vi "DIO_PWM_Encoder_SPI.vi"(0 "DIO.3:0.OUT":fxp<+,4,4> format="%.0b", 1 "DIO.3:0.DIR":fxp<+,4,4> format="%.0b", 2 "PWM.1:0.GROUP IN":T2 {"PWM.1.CNFG" format="%08b"; "PWM.0.CNFG" format="%08b"}, 3 "PWM.3:2.GROUP IN":T2 {"PWM.1.CNFG" format="%08b"; "PWM.0.CNFG" format="%08b"}, 4 "Encoder.0.GROUP IN":T1 {"ENC.STAT" format="%08b"}, 5 "Encoder.1.GROUP IN":T1 {"ENC.STAT" format="%08b"}, 6 "DIO0/PWM0/ENC0.A Refnum":refnum<k21>, 7 "DIO.3:0.Selector":fxp<+,8,8> format="%.0b", 8 "DIO1/PWM1/ENC0.B/SPI.CLK Refnum":refnum<k21>, 9 "SPI.GROUP IN":T3={"SPI.STAT"=0, "SPI.GO"=FALSE, "SPI.CNT"=19, "SPI.CNFG"=112, "SPI.DATI"=0, "SPI.DATO"=0} {"SPI.STAT" format="%08b"}, 10 "DIO2/PWM2/ENC1.A/SPI.MISO Refnum":refnum<k21>, 12 "DIO3/PWM3/ENC1.B/SPI.MOSI Refnum":refnum<k21>) -> (11 "SPI.GROUP OUT":T3={"SPI.STAT"=0, "SPI.GO"=FALSE, "SPI.CNT"=19, "SPI.CNFG"=112, "SPI.DATI"=0, "SPI.DATO"=0} {"SPI.STAT" format="%08b"}, 14 "IN 3:0":fxp<+,4,4> format="%02b", 16 "PWM.1:0.GROUP OUT":T2 {"PWM.1.CNFG" format="%08b"; "PWM.0.CNFG" format="%08b"}, 17 "PWM.3:2.GROUP OUT":T2 {"PWM.1.CNFG" format="%08b"; "PWM.0.CNFG" format="%08b"}, 18 "Encoder.0.GROUP OUT":T1 {"ENC.STAT" format="%08b"}, 19 "Encoder.1.GROUP OUT":T1 {"ENC.STAT" format="%08b"})   [LabVIEW 2021]
uses:
  Utilities/PWM Configuration Group.ctl
  Utilities/Encoder Configuration Group.ctl
  Utilities/Start Boolean.ctl
  Utilities/SPI Configuration Group.ctl
panel:
  # "This VI switches between the DIO functionality and the PWM/Encoder/SPI functionality for the specified FPGA I/O channels. Each bit has a selector which contains two-bits booleans.\n- If SELECT 0 is 00, DIO are enabled.\n- If SELECT 0 is 01, PWM enabled.\n- If SELECT 0 is 10, Encoder enabled.\n- If SELECT 0 is 11, SPI is enabled."
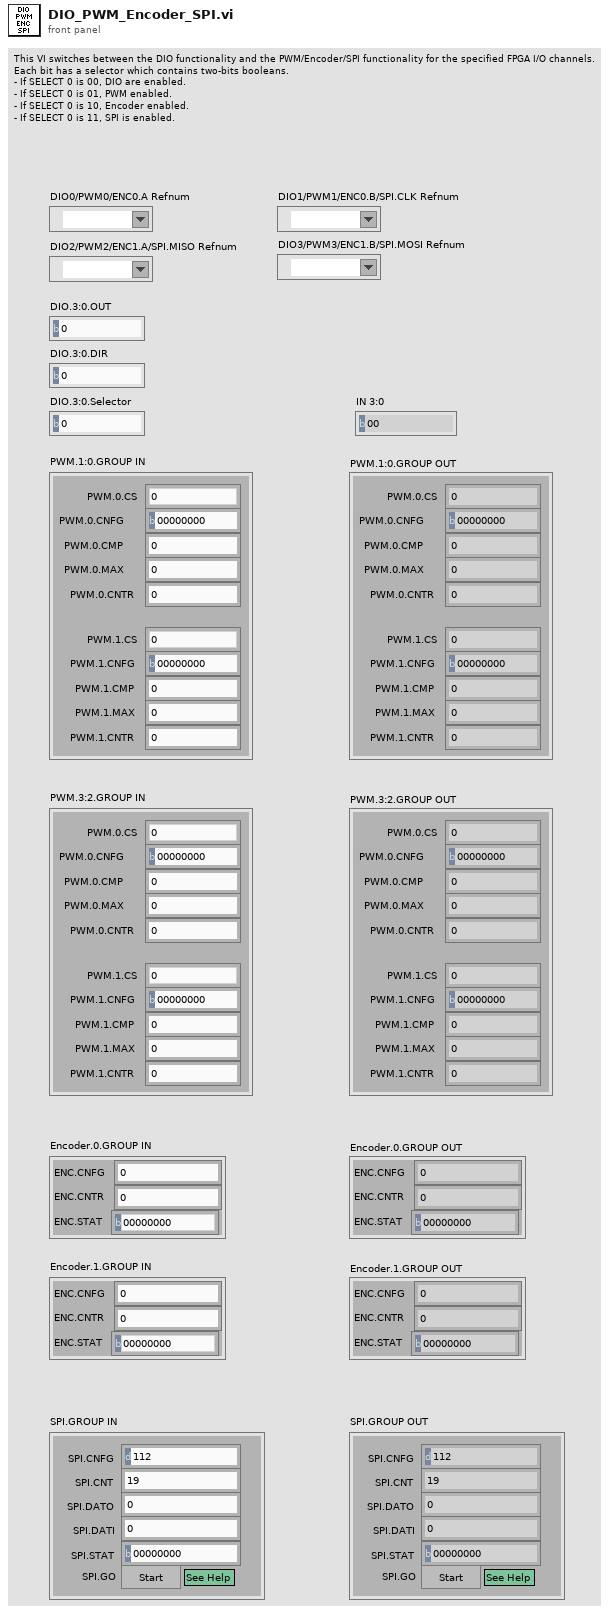
[diagram p1: front panel]
types:
  T1 = typedef "Encoder Configuration Group.ctl" = cluster{"ENC.CNFG":u8, "ENC.CNTR":u32, "ENC.STAT":u8}
  T2 = typedef "PWM Configuration Group.ctl" = cluster{"PWM.0.CS":u8, "PWM.0.CNFG":u8, "PWM.0.CMP":u16, "PWM.0.MAX":u16, "PWM.0.CNTR":u16, "PWM.1.CS":u8, "PWM.1.CNFG":u8, "PWM.1.CMP":u16, "PWM.1.MAX":u16, "PWM.1.CNTR":u16}
  T3 = typedef "SPI Configuration Group.ctl" = cluster{"SPI.STAT":u8, "SPI.GO":T4, "SPI.CNT":u16, "SPI.CNFG":u16, "SPI.DATI":u16, "SPI.DATO":u16}
  T4 = typedef "Start Boolean.ctl" = bool
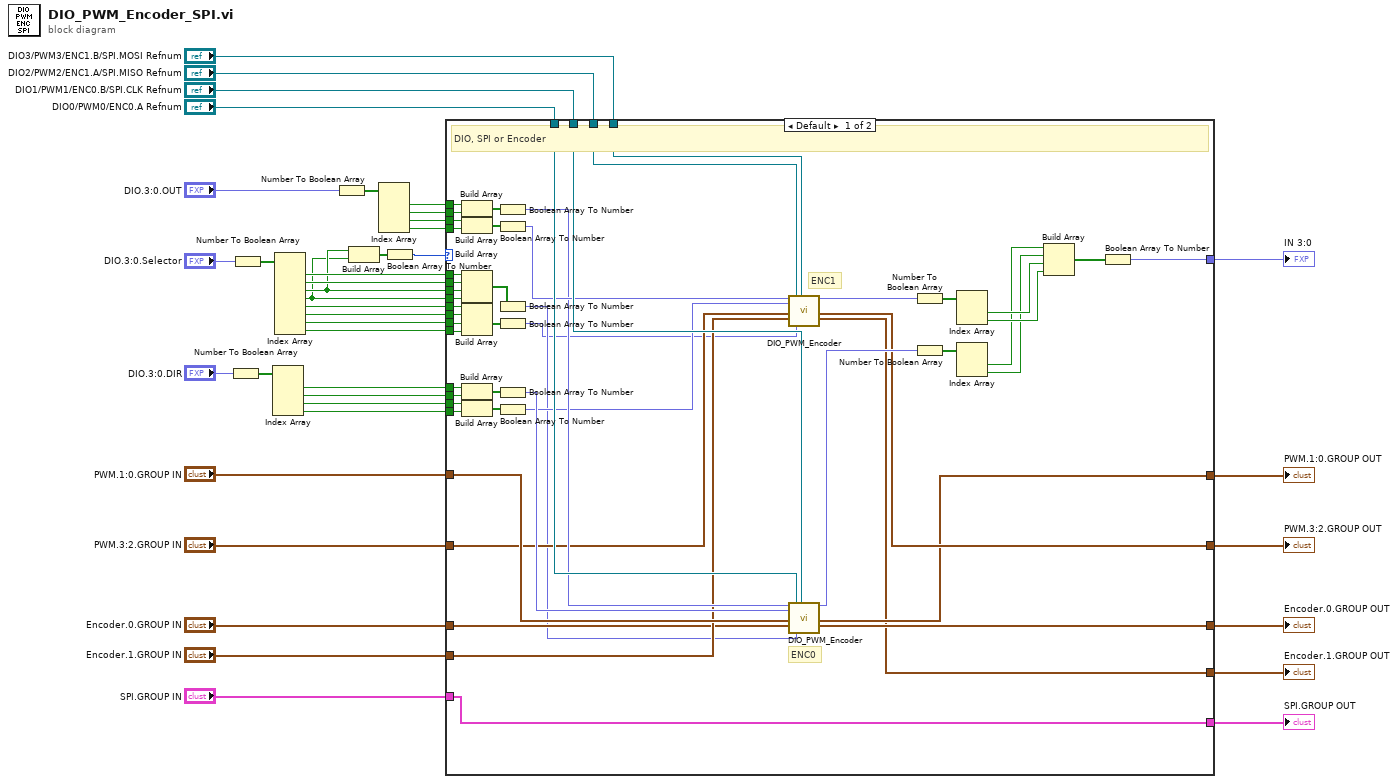
[diagram p0: block diagram]
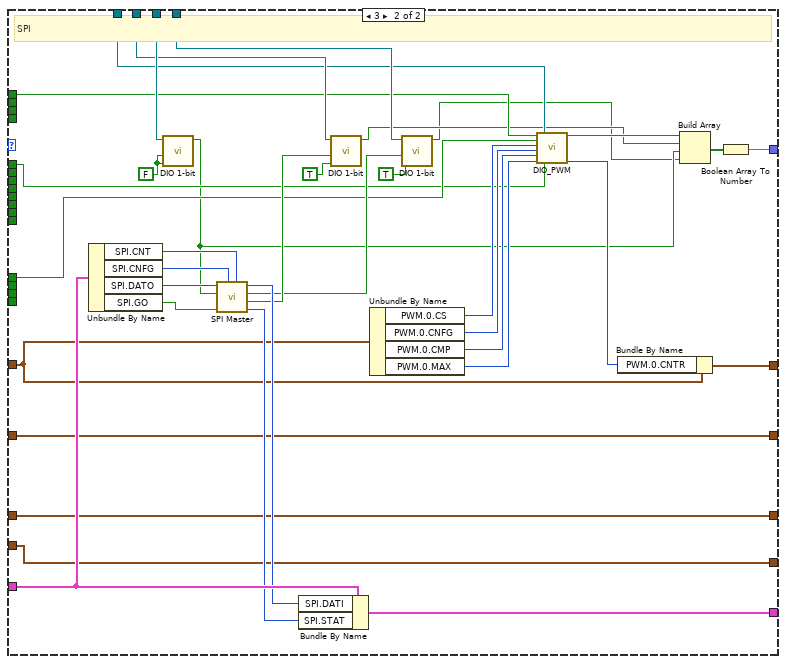
[diagram p2: hidden frame]
diagram:
  n1 = Number To Boolean Array(number="DIO.3:0.DIR") -> (Boolean array=w37:bool[])
  n2 = Number To Boolean Array(number="DIO.3:0.Selector") -> (Boolean array=w8:bool[])
  n3 = Index Array(array=w37) -> (element #1=w34:bool, element #2=w33:bool, element #3=w17:bool, element #4=w16:bool)  [unwired: 4 in]
  n4 = Index Array(array=w8) -> (element #1=w14:bool, element #2=w7:bool, element #3=w6:bool, element #4=w5:bool, element #5=w4:bool, element #6=w3:bool, element #7=w2:bool, element #8=w1:bool)  [unwired: 8 in]
  n5 = Number To Boolean Array(number="DIO.3:0.OUT") -> (Boolean array=w38:bool[])
  n6 = Build Array(w6, w5) -> (w26:bool[])
  n7 = Index Array(array=w38) -> (element #1=w31:bool, element #2=w32:bool, element #3=w23:bool, element #4=w24:bool)  [unwired: 4 in]
  n8 = Boolean Array To Number(Boolean array=w26) -> (number=w25:u8)
  n9 = case shown="Default" w25 {
    tunnel: w31 -> [w84 w105]
    tunnel: w32 -> [w83 _]
    tunnel: w34 -> [w74 w104]
    tunnel: w33 -> [w73 _]
    tunnel: "PWM.1:0.GROUP IN" -> [w68 w103]
    tunnel: "Encoder.0.GROUP IN" -> [w65 w100]
    tunnel: [w54 w101] -> w30
    tunnel: [w53 w100] -> w15
    tunnel: "SPI.GROUP IN" -> [w90 w122]
    tunnel: w24 -> [w79 _]
    tunnel: w23 -> [w80 _]
    tunnel: [w90 w107] -> w22
    tunnel: "DIO2/PWM2/ENC1.A/SPI.MISO Refnum" -> [w88 w119]
    tunnel: "DIO1/PWM1/ENC0.B/SPI.CLK Refnum" -> [w86 w115]
    tunnel: "DIO3/PWM3/ENC1.B/SPI.MOSI Refnum" -> [w87 w114]
    tunnel: "DIO0/PWM0/ENC0.A Refnum" -> [w85 w106]
    tunnel: w17 -> [w72 _]
    tunnel: w16 -> [w71 _]
    tunnel: w14 -> [w49 w99]
    tunnel: [w55 w98] -> w13
    tunnel: "PWM.3:2.GROUP IN" -> [w67 w98]
    tunnel: [w89 w92] -> w11
    tunnel: "Encoder.1.GROUP IN" -> [w66 w91]
    tunnel: [w52 w91] -> w9
    tunnel: w7 -> [w48 _]
    tunnel: w6 -> [w47 _]
    tunnel: w5 -> [w46 _]
    tunnel: w4 -> [w45 _]
    tunnel: w3 -> [w44 _]
    tunnel: w2 -> [w43 _]
    tunnel: w1 -> [w42 _]
    frame Default {
      # "ENC1"
      # "ENC0"
      # "DIO, SPI or Encoder"
      n10 = Build Array(w84, w83) -> (w82:bool[])
      n11 = Build Array(w80, w79) -> (w81:bool[])
      n12 = Build Array(w49, w48, w47, w46) -> (w51:bool[])
      n13 = Build Array(w45, w44, w43, w42) -> (w50:bool[])
      n14 = Build Array(w74, w73) -> (w75:bool[])
      n15 = Build Array(w72, w71) -> (w76:bool[])
      n16 = Boolean Array To Number(Boolean array=w82) -> (number=w77:fxp<+,2,2>)
      n17 = Boolean Array To Number(Boolean array=w81) -> (number=w78:fxp<+,2,2>)
      n18 = Boolean Array To Number(Boolean array=w51) -> (number=w41:fxp<+,4,4>)
      n19 = Boolean Array To Number(Boolean array=w50) -> (number=w40:fxp<+,4,4>)
      n20 = Boolean Array To Number(Boolean array=w75) -> (number=w70:fxp<+,2,2>)
      n21 = Boolean Array To Number(Boolean array=w76) -> (number=w69:fxp<+,2,2>)
      n22 = call "DIO_PWM_Encoder.vi"("DIO.1:0.OUT"=w78, "DIO.1:0.DIR"=w69, "PWM.GROUP IN"=w67, "Encoder.GROUP IN"=w66, "DIO0/PWM0/ENC.A Refnum"=w88, "DIO.1:0.Selector"=w40, "DIO1/PWM1/ENC.B Refnum"=w87) -> ("IN 1:0"=w63:fxp<+,2,2>, "PWM.GROUP OUT"=w55:T2, "Encoder.GROUP OUT"=w52:T1)  [unwired: 10 in]
      n23 = call "DIO_PWM_Encoder.vi"("DIO.1:0.OUT"=w77, "DIO.1:0.DIR"=w70, "PWM.GROUP IN"=w68, "Encoder.GROUP IN"=w65, "DIO0/PWM0/ENC.A Refnum"=w85, "DIO.1:0.Selector"=w41, "DIO1/PWM1/ENC.B Refnum"=w86) -> ("IN 1:0"=w61:fxp<+,2,2>, "PWM.GROUP OUT"=w54:T2, "Encoder.GROUP OUT"=w53:T1)  [unwired: 10 in]
      n24 = Number To Boolean Array(number=w63) -> (Boolean array=w64:bool[])
      n25 = Number To Boolean Array(number=w61) -> (Boolean array=w62:bool[])
      n26 = Index Array(array=w64) -> (element #1=w60:bool, element #2=w59:bool)  [unwired: 2 in]
      n27 = Index Array(array=w62) -> (element #1=w57:bool, element #2=w58:bool)  [unwired: 2 in]
      n28 = Build Array(w57, w58, w60, w59) -> (w56:bool[])
      n29 = Boolean Array To Number(Boolean array=w56) -> (number=w89:fxp<+,4,4>)
    }
    frame 3 {
      w118 = FALSE ("DIR")
      # "SPI"
      n30 = Unbundle By Name(w122) -> ("SPI.CNT"=w126:u16, "SPI.CNFG"=w125:u16, "SPI.DATO"=w124:u16, "SPI.GO"=w123:T4)
      n31 = call "DIO 1-bit.vi"("DIR"=w118, "OUT"=w118, "DIO Refnum"=w119) -> ("IN"=w95:bool)  [unwired: 8 in]
      n32 = call "SPI Master.vi"("Count"=w126, "Configuration"=w125, "Start?"=w123, "MISO"=w95, "Data Out"=w124) -> ("Status"=w120:u8, "SCLK"=w113:bool, "MOSI"=w112:bool, "Data In"=w121:u16)  [unwired: 3 in]
      n33 = Bundle By Name(cluster=w122, "SPI.DATI"=w121, "SPI.STAT"=w120) -> (w107:T3)
      n34 = call "DIO 1-bit.vi"("DIR"=TRUE, "OUT"=w113, "DIO Refnum"=w115) -> ("IN"=w96:bool)  [unwired: 8 in]
      n35 = Unbundle By Name(w103) -> ("PWM.0.CS"=w108:u8, "PWM.0.CNFG"=w109:u8, "PWM.0.CMP"=w110:u16, "PWM.0.MAX"=w111:u16)
      n36 = call "DIO 1-bit.vi"("DIR"=TRUE, "OUT"=w112, "DIO Refnum"=w114) -> ("IN"=w94:bool)  [unwired: 8 in]
      n37 = call "DIO_PWM.vi"("DIO.OUT"=w105, "DIO.DIR"=w104, "PWM.CS"=w108, "PWM.CNFG"=w109, "PWM.CMP"=w110, "PWM.MAX"=w111, "DIO/PWM"=w106, "SELECT"=w99) -> ("DIO.IN"=w97:bool, "PWM.CNTR"=w102:u16)  [unwired: 10 in]
      n38 = Bundle By Name(cluster=w103, "PWM.0.CNTR"=w102) -> (w101:T2)
      n39 = Build Array(w97, w96, w95, w94) -> (w93:bool[])
      n40 = Boolean Array To Number(Boolean array=w93) -> (number=w92:fxp<+,4,4>)
    }
  }
  "IN 3:0" <- w11
  "Encoder.0.GROUP OUT" <- w15
  "PWM.1:0.GROUP OUT" <- w30
  "SPI.GROUP OUT" <- w22
  "PWM.3:2.GROUP OUT" <- w13
  "Encoder.1.GROUP OUT" <- w9
